vi "CPT-Compute PTC.vi"(0 "Response":dbl[][](array[numeric]), 7 "Response":T2, 9 "Fs (Hz)":dbl, 11 "error in (no error)":errorcluster) -> (6 "data":T1, 15 "error out":errorcluster)   [LabVIEW 2020]
uses:
  Typedefs/PTC-Response.ctl
  Common VIs/Typedefs/CAL-Data.ctl
  epl-vi-lib/Utility VIs/Math VIs/FFT x(t) to dB,Degrees (2D).vi
panel:
  out "Frequency":dbl[](array[numeric])
  out "PTC Phase":dbl[](array[numeric])
  out "PTC Mag":dbl[](array[numeric])
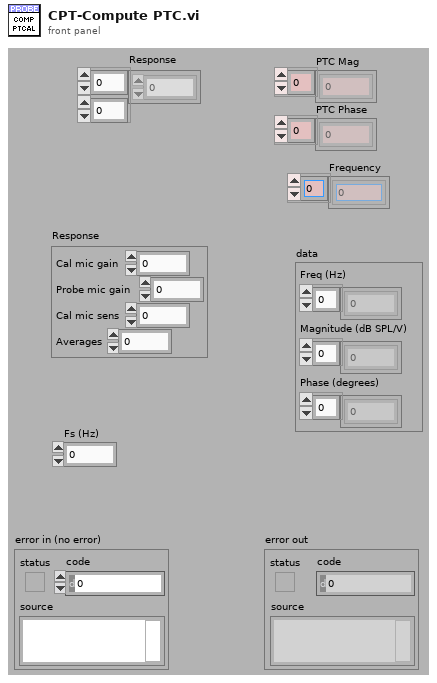
[diagram p1: front panel]
types:
  T1 = typedef "CAL-Data.ctl" = cluster{"Freq (Hz)":dbl[], "Magnitude (dB SPL/V)":dbl[], "Phase (degrees)":dbl[]}
  T2 = typedef "PTC-Response.ctl" = cluster{"Cal mic gain":dbl, "Probe mic gain":dbl, "Cal mic sens":dbl, "Averages":i32}
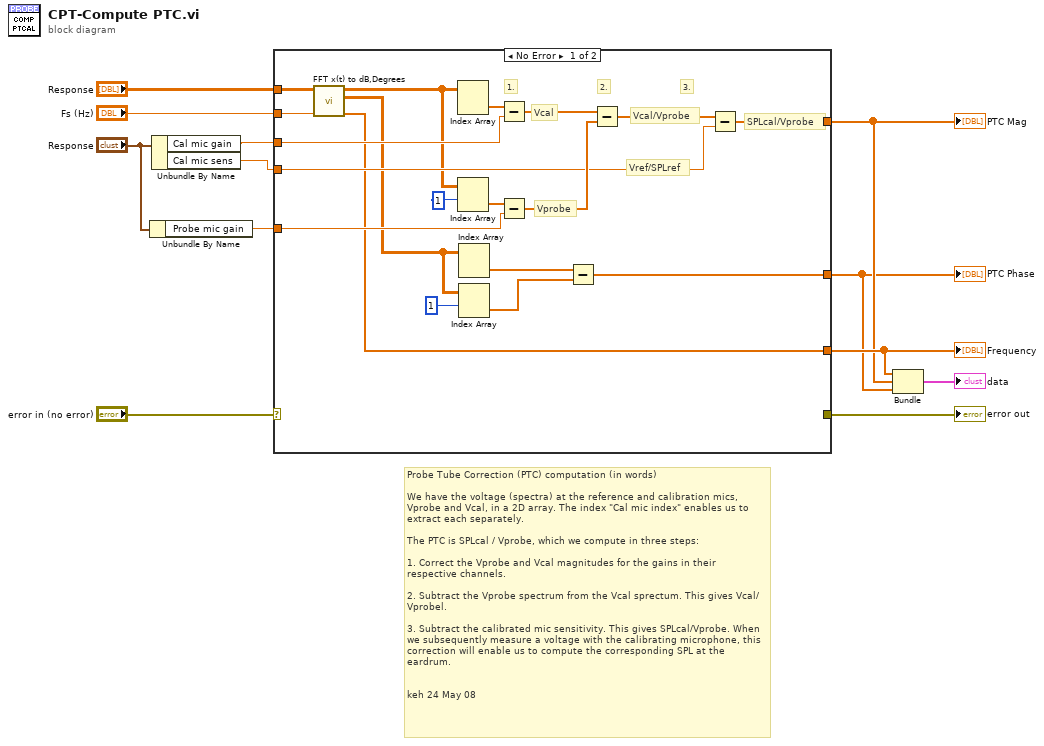
[diagram p0: block diagram]
diagram:
  # "Probe Tube Correction (PTC) computation (in words)\n\nWe have the voltage (spectra) at the reference and calibration mics, Vprobe and Vcal, in a 2D array. The index \"Cal mic index\" enables us to extract each separately. \n\nThe PTC is SPLcal / Vprobe, which we compute in three steps:\n\n1. Correct the Vprobe and Vcal magnitudes for the gains in their respective channels.\n\n2. Subtract the Vprobe spectrum from the Vcal sprectum. This gives Vcal/Vprobel.\n\n3. Subtract the calibrated mic sensitivity. This gives SPLcal/Vprobe. When we subsequently measure a voltage with the calibrating microphone, this correction will enable us to compute the corresponding SPL at the eardrum.\n\n\nkeh 24 May 08"
  n1 = Unbundle By Name("Response") -> ("Probe mic gain"=w6:dbl)
  n2 = Unbundle By Name("Response") -> ("Cal mic gain"=w9:dbl, "Cal mic sens"=w8:dbl)
  n3 = case shown="No Error" "error in (no error)" {
    selector: "error in (no error)" -> [_ w32]
    tunnel: "Response" -> [w19 _]
    tunnel: [w20 _] -> w4
    tunnel: [w30 _] -> w3
    tunnel: [w14 _] -> w5
    tunnel: [_ w32] -> w10
    tunnel: w9 -> [w26 _]
    tunnel: w6 -> [w24 _]
    tunnel: w8 -> [w21 _]
    tunnel: "Fs (Hz)" -> [w13 _]
    frame No Error {
      # "Vref/SPLref"
      # "SPLcal/Vprobe"
      # "Vcal/Vprobe"
      # "Vprobe"
      # "Vcal"
      # "3."
      # "2."
      # "1."
      n4 = call-poly "FFT x(t) to dB,Degrees.vi"("Fs (Hz)"=w13, "X(t)"=w19) -> ("Freq (Hz)"=w14:dbl[], "+Freq Phase of FFT (degrees)"=w16:dbl[][], "+Freq. Mag of FFT (dB rms)"=w18:dbl[][])  [unwired: 7 in]
      n5 = Index Array(array=w18) -> (element=w27:dbl[])  [unwired: 2 in]
      n6 = Index Array(array=w18, index (row)=1 ("x")) -> (element=w25:dbl[])  [unwired: 1 in]
      n7 = Index Array(array=w16) -> (element=w31:dbl[])  [unwired: 2 in]
      n8 = Index Array(array=w16, index (row)=1 ("x")) -> (element=w29:dbl[])  [unwired: 1 in]
      n9 = Subtract(x=w27, y=w26) -> (x-y=w28:dbl[])
      n10 = Subtract(x=w25, y=w24) -> (x-y=w23:dbl[])
      n11 = Subtract(x=w31, y=w29) -> (x-y=w30:dbl[])
      n12 = Subtract(x=w28, y=w23) -> (x-y=w22:dbl[])
      n13 = Subtract(x=w22, y=w21) -> (x-y=w20:dbl[])
    }
    frame Error {
    }
  }
  "PTC Mag" <- w4
  "PTC Phase" <- w3
  "Frequency" <- w5
  "error out" <- w10
  n14 = Bundle("Freq (Hz)"=w5, w4, w3) -> (→"data":cluster{"Freq (Hz)":dbl[], dbl[], dbl[]})  [unwired: 1 in]
